vi "Formatting Duration.vi"(8 "error in":errorcluster, 10 "Error Input Values":variant, 11 "Error Code":i32) -> (0 "Generated Error":errorcluster, 3 "Formatting Generation Duration [ms]":dbl)   [LabVIEW 2021]
doc: "Measure the duration of <b>Generate Error</b> function with specific formatting inputs that are avaiable also as an inputs to this VI. The resulting duration is returned at <b>Formatting Generation Duration [ms]</b>"
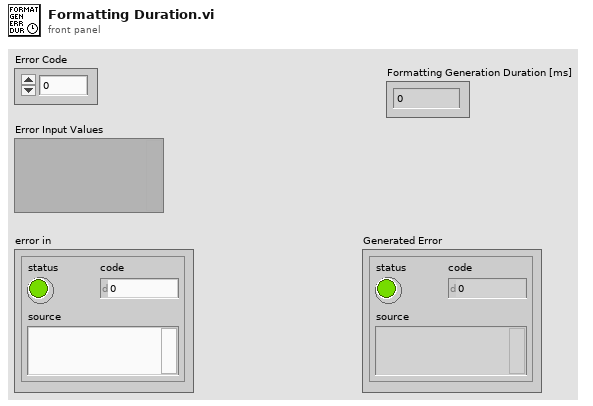
[diagram p1: front panel]
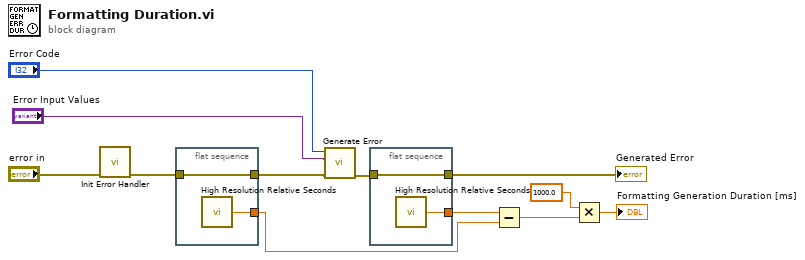
[diagram p0: block diagram]
diagram:
  n1 = call "Init Error Handler.vi"("error in"="error in") -> ("error out"=w12:errorcluster)  [unwired: 10 in]
  n2 = flat-sequence {
    tunnel: [w14] -> w3
    tunnel: w12 -> [w14]
    tunnel: [w13] -> w7
    frame #0 {
      n3 = call <vilib>:"High Resolution Relative Seconds.vi"() -> ("relative seconds"=w13:dbl)
    }
  }
  n4 = call "Generate Error.vi"("error in"=w3, "Error Input Values"="Error Input Values", "Error Code"="Error Code") -> ("Generated Error"=w4:errorcluster)  [unwired: 8 in]
  n5 = flat-sequence {
    tunnel: [w16] -> w5
    tunnel: w4 -> [w16]
    tunnel: [w15] -> w8
    frame #0 {
      n6 = call <vilib>:"High Resolution Relative Seconds.vi"() -> ("relative seconds"=w15:dbl)
    }
  }
  n7 = Subtract(x=w8, y=w7) -> (x-y=w10:dbl)
  n8 = Multiply(x=1000.0, y=w10) -> (x*y=→"Formatting Generation Duration [ms]":dbl)
  "Generated Error" <- w5
